vi "Forums.vi"() -> ()   [LabVIEW 2026, in "LMH-LINX.lvlib"]
uses:
  <vilib>/MakerHub/LINX/LMH-LINX.lvlib
  <vilib>/Platform/browser.llb/Open URL in Default Browser (string).vi
  <vilib>/MakerHub/Toolbox/LMH-Toolbox.lvlib
panel:
  out "Error Out":errorcluster
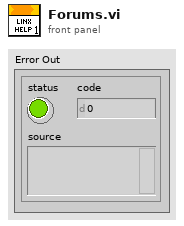
[diagram p1: front panel]
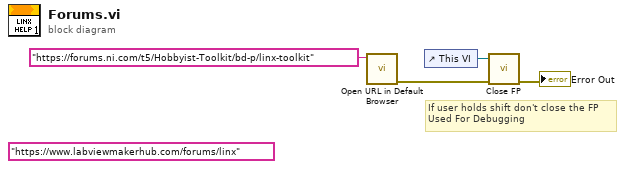
[diagram p0: block diagram]
diagram:
  (unwired) "https://www.labviewmakerhub.com/forums/linx" ("URL")
  # "If user holds shift don't close the FP\nUsed For Debugging"
  n1 = call-poly <vilib>:"Open URL in Default Browser.vi"("URL"="https://forums.ni.com/t5/Hobbyist-Toolkit/bd-p/linx-toolkit") -> ("error out"=w1:errorcluster)  [unwired: 5 in, 1 out]
  n2 = control-ref of="This VI"() -> (w2:refnum<vi>)
  n3 = call <vilib>:"Close FP.vi"("Error In"=w1, "VI Ref"=w2) -> ("Error Out"=→"Error Out":errorcluster)  [unwired: 9 in]
